vi "Front of Rocket From Ready Feeder.vi"() -> (4 "path":cluster{"X":dbl, "Y":dbl}[](array[cluster])=[{"X"=118.0, "Y"=82.0}, {"X"=118.95573916314487, "Y"=81.7142151110502}, {"X"=119.9112889589267, "Y"=81.42818959606394}, {"X"=120.86644186709641, "Y"=81.14170784456527}, {"X"=121.82095500191464, "Y"=80.8545207528199}, {"X"=122.77456839209741, "Y"=80.56631700439428}, {"X"=123.726975543945, "Y"=80.27674214273533}, {"X"=124.67779389465163, "Y"=79.98538333403357}, {"X"=125.62655326893304, "Y"=79.69172926636989}, {"X"=126.572682887376, "Y"=79.39513838103505}, {"X"=127.51548174962639, "Y"=79.0948147862806}, {"X"=128.45407460540636, "Y"=78.78977329795943}, {"X"=129.38736073320499, "Y"=78.47878457907608}, {"X"=130.31395643926723, "Y"=78.16030370732027}, {"X"=131.23212545443386, "Y"=77.83238616687454}, {"X"=132.1396896678511, "Y"=77.49258815219099}, {"X"=133.0339142103294, "Y"=77.13784209836672}, {"X"=133.91136206209498, "Y"=76.76429707135958}, {"X"=134.76771224033126, "Y"=76.36711488454004}, {"X"=135.59753264884552, "Y"=75.94021301709624}, {"X"=136.4148505017556, "Y"=75.4698231924859}, {"X"=137.22222143075993, "Y"=74.9648467556594}, {"X"=138.0216783124796, "Y"=74.43236422575896}, {"X"=138.81483754115675, "Y"=73.87800911804504}, {"X"=139.60298333391162, "Y"=73.30626478782413}, {"X"=140.38713502049174, "Y"=72.72069991143931}, {"X"=141.16810101928868, "Y"=72.12415552113453}, {"X"=141.9465221205076, "Y"=71.51889401796474}, {"X"=142.72290594419815, "Y"=70.90671827866095}, {"X"=143.4976540315866, "Y"=70.28906701066101}, {"X"=144.27108285061033, "Y"=69.66709103831158}, {"X"=145.04344009347295, "Y"=69.04171406851535}, {"X"=145.81491546528602, "Y"=68.41368255903322}, {"X"=146.58565989671, "Y"=67.78359676265896}, {"X"=147.35575287171008, "Y"=67.15197423377705}, {"X"=148.12532373221526, "Y"=66.51918424646601}, {"X"=148.89431846524718, "Y"=65.88565443494305}, {"X"=149.66283732607528, "Y"=65.2516336981667}, {"X"=150.43083972308645, "Y"=64.61742860060318}, {"X"=151.19825066364893, "Y"=63.98334639957007}, {"X"=151.96502223897846, "Y"=63.349658348645626}, {"X"=152.7310689648106, "Y"=62.71665704314593}, {"X"=153.4962352739256, "Y"=62.08469517015696}, {"X"=154.26031610247122, "Y"=61.45418442345999}, {"X"=155.02306792662387, "Y"=60.82559931877291}, {"X"=155.78418706764904, "Y"=60.199506741166836}, {"X"=156.54327670955732, "Y"=59.57660846426381}, {"X"=157.29982232098143, "Y"=58.95778233022209}, {"X"=158.05317306549708, "Y"=58.34412325219512}, {"X"=158.80251577005876, "Y"=57.73699465188104}, {"X"=159.54683263200243, "Y"=57.13809912865052}, {"X"=160.2848424677819, "Y"=56.549571457288785}, {"X"=161.01492847905695, "Y"=55.97409463395153}, {"X"=161.73505245076166, "Y"=55.41504202149926}, {"X"=162.44265024140935, "Y"=54.87665307226513}, {"X"=163.1735416287964, "Y"=54.331775326204486}, {"X"=163.9229565815191, "Y"=53.78173996112071}, {"X"=164.6871020397987, "Y"=53.227604728564195}, {"X"=165.4629602301617, "Y"=52.67021106349252}, {"X"=166.24812826110352, "Y"=52.110229733758445}, {"X"=167.04069139609203, "Y"=51.548196655201416}, {"X"=167.83912320057857, "Y"=50.984540667276555}, {"X"=168.6422061389889, "Y"=50.41960546784218}, {"X"=169.4489702497214, "Y"=49.85366564642543}, {"X"=170.25863424170058, "Y"=49.28694640068653}, {"X"=171.07058637482402, "Y"=48.719620139332136}, {"X"=171.8843055748802, "Y"=48.15184703877353}, {"X"=172.69939771616944, "Y"=47.583742590545555}, {"X"=173.51551806504807, "Y"=47.015415710212245}, {"X"=174.3323752802064, "Y"=46.446970398217125}, {"X"=175.14972583736272, "Y"=45.87849502533809}, {"X"=175.9673520727771, "Y"=45.31007477866971}, {"X"=176.78504692981505, "Y"=44.74180346005197}, {"X"=177.60260655960224, "Y"=44.17378365571832}, {"X"=178.41982252526935, "Y"=43.60612722019072}, {"X"=179.23647002823668, "Y"=43.03896303004192}, {"X"=180.05229361866736, "Y"=42.47244769798032}, {"X"=180.8669924736217, "Y"=41.906774526422595}, {"X"=181.6802052647786, "Y"=41.34218157294263}, {"X"=182.49149269539075, "Y"=40.77896242885303}, {"X"=183.30031532302328, "Y"=40.2174818281647}, {"X"=184.1060049413875, "Y"=39.65819603138085}, {"X"=184.90772866923282, "Y"=39.101677508094475}, {"X"=185.70444387377512, "Y"=38.54864509752359}, {"X"=186.49484536082474, "Y"=38.0}], 6 "Reverse Path?":bool)   [LabVIEW 2018]
uses:
  AutonBuilder/Typedef/Data Point.ctl
panel:
  in  "Data Points":T1[](array[typedef])=[{"X"=118.0, "Y"=82.0, "Theta"=0.0, "Speed %"=0.0, "Disabled?"=FALSE}, {"X"=135.83505154639175, "Y"=76.76655052264809, "Theta"=0.0, "Speed %"=0.0, "Disabled?"=FALSE}, {"X"=162.0, "Y"=55.0, "Theta"=0.0, "Speed %"=0.0, "Disabled?"=FALSE}, {"X"=186.49484536082474, "Y"=38.0, "Theta"=0.0, "Speed %"=0.0, "Disabled?"=FALSE}]
  out "Graph":cluster{dbl[], dbl[]}[](graph)=[{[98.5, 132.0, 132.0, 98.5, 98.5], [96.25, 96.25, 67.75, 67.75, 96.25]}, {[118.0, 135.83505154639175, 162.0, 186.49484536082474], [82.0, 76.76655052264809, 55.0, 38.0]}, {[118.0, 118.95573916314487, 119.9112889589267, 120.86644186709641, 121.82095500191464, 122.77456839209741, 123.726975543945, 124.67779389465163, 125.62655326893304, 126.572682887376, 127.51548174962639, 128.45407460540636, 129.38736073320499, 130.31395643926723, 131.23212545443386, 132.1396896678511, 133.0339142103294, 133.91136206209498, 134.76771224033126, 135.59753264884552, 136.4148505017556, 137.22222143075993, 138.0216783124796, 138.81483754115675, 139.60298333391162, 140.38713502049174, 141.16810101928868, 141.9465221205076, 142.72290594419815, 143.4976540315866, 144.27108285061033, 145.04344009347295, 145.81491546528602, 146.58565989671, 147.35575287171008, 148.12532373221526, 148.89431846524718, 149.66283732607528, 150.43083972308645, 151.19825066364893, 151.96502223897846, 152.7310689648106, 153.4962352739256, 154.26031610247122, 155.02306792662387, 155.78418706764904, 156.54327670955732, 157.29982232098143, 158.05317306549708, 158.80251577005876, 159.54683263200243, 160.2848424677819, 161.01492847905695, 161.73505245076166, 162.44265024140935, 163.1735416287964, 163.9229565815191, 164.6871020397987, 165.4629602301617, 166.24812826110352, 167.04069139609203, 167.83912320057857, 168.6422061389889, 169.4489702497214, 170.25863424170058, 171.07058637482402, 171.8843055748802, 172.69939771616944, 173.51551806504807, 174.3323752802064, 175.14972583736272, 175.9673520727771, 176.78504692981505, 177.60260655960224, 178.41982252526935, 179.23647002823668, 180.05229361866736, 180.8669924736217, 181.6802052647786, 182.49149269539075, 183.30031532302328, 184.1060049413875, 184.90772866923282, 185.70444387377512, 186.49484536082474], [82.0, 81.7142151110502, 81.42818959606394, 81.14170784456527, 80.8545207528199, 80.56631700439428, 80.27674214273533, 79.98538333403357, 79.69172926636989, 79.39513838103505, 79.0948147862806, 78.78977329795943, 78.47878457907608, 78.16030370732027, 77.83238616687454, 77.49258815219099, 77.13784209836672, 76.76429707135958, 76.36711488454004, 75.94021301709624, 75.4698231924859, 74.9648467556594, 74.43236422575896, 73.87800911804504, 73.30626478782413, 72.72069991143931, 72.12415552113453, 71.51889401796474, 70.90671827866095, 70.28906701066101, 69.66709103831158, 69.04171406851535, 68.41368255903322, 67.78359676265896, 67.15197423377705, 66.51918424646601, 65.88565443494305, 65.2516336981667, 64.61742860060318, 63.98334639957007, 63.349658348645626, 62.71665704314593, 62.08469517015696, 61.45418442345999, 60.82559931877291, 60.199506741166836, 59.57660846426381, 58.95778233022209, 58.34412325219512, 57.73699465188104, 57.13809912865052, 56.549571457288785, 55.97409463395153, 55.41504202149926, 54.87665307226513, 54.331775326204486, 53.78173996112071, 53.227604728564195, 52.67021106349252, 52.110229733758445, 51.548196655201416, 50.984540667276555, 50.41960546784218, 49.85366564642543, 49.28694640068653, 48.719620139332136, 48.15184703877353, 47.583742590545555, 47.015415710212245, 46.446970398217125, 45.87849502533809, 45.31007477866971, 44.74180346005197, 44.17378365571832, 43.60612722019072, 43.03896303004192, 42.47244769798032, 41.906774526422595, 41.34218157294263, 40.77896242885303, 40.2174818281647, 39.65819603138085, 39.101677508094475, 38.54864509752359, 38.0]}, {[126.10013206929261, 114.87331144513882, 115.82496325782363, 116.77257514583421, 117.71532165090885, 118.65205209155243, 119.58169832407744, 120.50279043567588, 121.41318516451578, 122.31014980301123, 123.1903555222424, 124.04961361286838, 124.88250558258584, 125.6820432181841, 126.43933134314666, 127.14312428812163, 127.7792087227776, 128.3296393001962, 128.77195544449881, 129.07866805415483, 129.30673089936005, 129.6657597525321, 130.12222066438255, 130.6514647388213, 131.23544733877966, 131.86090626836966, 132.51802193810374, 133.19946344683018, 133.89971426188924, 134.6145922655976, 135.34090390637405, 136.07619257760143, 136.81855327501472, 137.56650893861269, 138.31886728949817, 139.07480107201408, 139.83344463830304, 140.59444254639024, 141.357249293099, 142.12154968805226, 142.8871793983201, 143.65397341052767, 144.42180159288847, 145.19062599987322, 145.96048975304802, 146.73148958007735, 147.50378370513633, 148.27763125267788, 149.05344011444492, 149.8318195113156, 150.61365754557235, 151.40025613068482, 152.1935636750775, 152.99656819771857, 153.81397097082095, 154.65649809091272, 155.491395753969, 156.32153002351905, 157.14864895937367, 157.97383178800476, 158.79775180523976, 159.62083229869884, 160.44333968072553, 161.26544227099876, 162.08723661599387, 162.90879475573897, 163.73011863775199, 164.55125647258473, 165.37214358699427, 166.19280729596576, 167.01317884693708, 167.83318616496757, 168.65277819408996, 169.47185847827058, 170.29027797187283, 171.10786690396327, 171.92443236904614, 172.73972382325786, 173.55340661496777, 174.3650550564733, 175.17414533359292, 175.98002990982886, 176.78189424470537, 177.57870298895617, 178.36915150196302], [70.27607742860704, 68.06151267060801, 67.77665333582918, 67.49243111396369, 67.20877875074801, 66.9256660172991, 66.64299075984562, 66.36070549866659, 66.07886662779606, 65.79759037763769, 65.51704681370148, 65.2375327686148, 64.95958415627221, 64.68410691770802, 64.41256408881364, 64.14729555869238, 63.89206653635855, 63.65297101297399, 63.43988005085542, 63.26871332700082, 63.119230667508006, 62.88335732324776, 62.572302300713154, 62.19803289845926, 61.77167154097876, 61.30291013992544, 60.799905793702386, 60.26938449269012, 59.716821561656126, 59.146638475479634, 58.562389150195955, 57.966924138720024, 57.36253025072361, 56.75103513831023, 56.13393452727705, 55.51234366539168, 54.887333404340296, 54.259513060192376, 53.62959638906845, 52.99808357159903, 52.36533909981152, 51.73172025232108, 51.09755935737761, 50.46313254282382, 49.82868262145149, 49.194454801329705, 48.56070785546091, 47.9277067036897, 47.2957158190061, 46.6649980553601, 46.035807343834875, 45.40835852427885, 44.78275767203708, 44.15887069376451, 43.53608897494978, 42.90713225196387, 42.293864526066464, 41.69158700837849, 41.09719382111156, 40.50856959930934, 39.924236619931165, 39.34314063755156, 38.764516931088636, 38.187802205536734, 37.61258299865922, 37.0385389579246, 36.46545600499549, 35.893135494479345, 35.321487708459294, 34.75039256408442, 34.1798154813641, 33.609739527736544, 33.0401495081549, 32.4710730450127, 31.90258052039323, 31.33476244870991, 30.767731917282966, 30.20164726163759, 29.636727984745672, 29.073258208226832, 28.511591802076076, 27.952170668923905, 27.395554541665135, 26.842457200826317, 26.293779460814136]}, {[109.89986793070739, 123.03816688115091, 123.99761466002978, 124.96030858835861, 125.92658835292043, 126.89708469264238, 127.87225276381257, 128.85279735362738, 129.83992137335028, 130.83521597174078, 131.8406079770104, 132.85853559794432, 133.89221588382412, 134.94586966035035, 136.02491956572106, 137.13625504758056, 138.28861969788122, 139.49308482399377, 140.7634690361637, 142.1163972435362, 143.52297010415117, 144.77868310898776, 145.92113596057663, 146.9782103434922, 147.97051932904358, 148.91336377261382, 149.81818010047363, 150.69358079418504, 151.54609762650705, 152.3807157975756, 153.2012617948466, 154.01068760934447, 154.81127765555732, 155.60481085480734, 156.392638453922, 157.17584639241645, 157.95519229219133, 158.7312321057603, 159.5044301530739, 160.27495163924561, 161.04286507963684, 161.8081645190935, 162.57066895496274, 163.33000620506922, 164.0856461001997, 164.83688455522073, 165.5827697139783, 166.322013389285, 167.05290601654923, 167.77321202880194, 168.48000771843252, 169.169428804879, 169.83629328303638, 170.47353670380474, 171.07132951199776, 171.69058516668005, 172.3545174090692, 173.05267405607836, 173.77727150094975, 174.52242473420227, 175.2836309869443, 176.0574141024583, 176.8410725972523, 177.63249822844406, 178.43003186740728, 179.23237799390907, 180.0384925120084, 180.84753895975416, 181.65889254310187, 182.47194326444705, 183.28627282778837, 184.1015179805866, 184.91731566554014, 185.7333546409339, 186.54936707866588, 187.3650731525101, 188.18015486828858, 188.99426112398555, 189.80700391458944, 190.6179303343082, 191.42648531245365, 192.23197997294616, 193.03356309376028, 193.83018475859407, 194.62053921968646], [93.72392257139296, 95.36691755149238, 95.07972585629871, 94.79098457516686, 94.50026275489178, 94.20696799148946, 93.91049352562504, 93.61006116940055, 93.30459190494372, 92.99268638443242, 92.6725827588597, 92.34201382730406, 91.99798500187994, 91.63650049693251, 91.25220824493545, 90.8378807456896, 90.38361766037488, 89.87562312974516, 89.29434971822467, 88.61171270719166, 87.8204157174638, 87.04633618807102, 86.29242615080477, 85.55798533763083, 84.84085803466951, 84.13848968295318, 83.44840524856667, 82.76840354323936, 82.09661499566576, 81.4314955458424, 80.77179292642721, 80.11650399831066, 79.46483486734283, 78.81615838700769, 78.17001394027706, 77.52602482754034, 76.8839754655458, 76.24375433614102, 75.6052608121379, 74.9686092275411, 74.33397759747973, 73.70159383397078, 73.07183098293632, 72.44523630409617, 71.82251601609433, 71.20455868100397, 70.59250907306671, 69.98785795675447, 69.39253068538413, 68.80899124840198, 68.24039091346617, 67.69078439029872, 67.16543159586598, 66.67121334923401, 66.21721716958048, 65.7564184004451, 65.26961539617496, 64.7636224487499, 64.24322830587349, 63.71188986820755, 63.17215669047167, 62.625940697001546, 62.07469400459573, 61.51952908731413, 60.96130980271384, 60.40070132073967, 59.838238072551576, 59.274349686611764, 58.7093437119652, 58.14354823234983, 57.57717456931208, 57.01041002960287, 56.44345741194904, 55.87649426642393, 55.309673919988214, 54.74316361137393, 54.17716347867768, 53.6119017912076, 53.04763516113958, 52.48466664947922, 51.923371854253325, 51.36422139383779, 50.807800474523816, 50.25483299422086, 49.706220539185864]}, {[], []}, {[], []}, {[], []}, {[], []}, {[], []}, {[], []}, {[], []}, {[], []}, {[], []}, {[], []}, {[], []}, {[], []}, {[], []}, {[], []}, {[], []}, {[], []}, {[], []}, {[], []}, {[], []}, {[], []}]
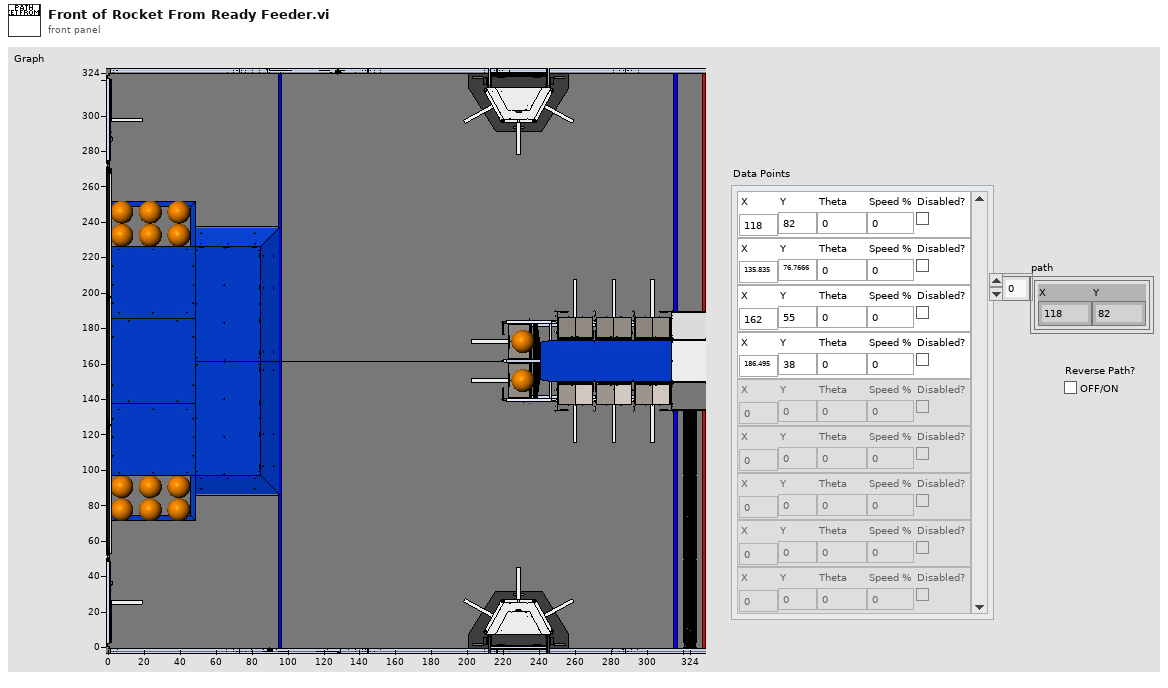
[diagram p1: front panel]
types:
  T1 = typedef "Data Point.ctl" = cluster{"X":dbl, "Y":dbl, "Theta":dbl, "Speed %":dbl, "Disabled?":bool}
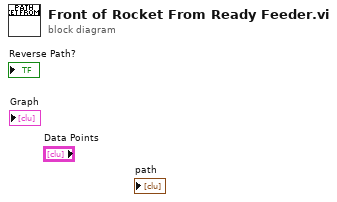
[diagram p0: block diagram]
diagram:
